vi "FuncImg-Event handler-Groups mouse up.vi"(9 "Coords":T1) -> ()   [LabVIEW 2017]
uses:
  <vilib>/Utility/miscctls.llb/LVPoint32TypeDef.ctl
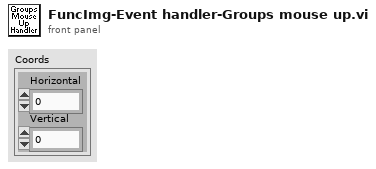
[diagram p1: front panel]
types:
  T1 = typedef "LVPoint32TypeDef.ctl" = cluster{"Horizontal":i32, "Vertical":i32}
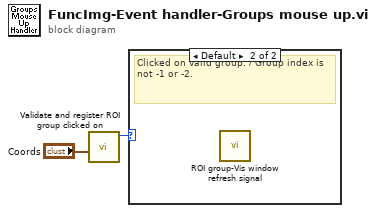
[diagram p0: block diagram]
diagram:
  n1 = call "Validate and register ROI group clicked on.vi"("Coords"="Coords") -> ("Index of group clicked on"=w2:i16)  [unwired: 8 in, 2 out]
  n2 = case shown="Default" w2 {
    frame -2, -1 {
      # "Invalid group index"
    }
    frame Default {
      # "Clicked on valid group. / Group index is not -1 or -2."
      n3 = call "ROI group-Vis window refresh signal.vi"() -> ()  [unwired: 11 in, 1 out]
    }
  }
